vi "niFpgaFFTSimModelStreamingCoreWrapper.vi"(0 "real data in":fxp<+/-,16,1>, 1 "reset":bool, 5 "imaginary data in":fxp<+/-,16,1>, 7 "input valid":bool=TRUE, 12 "ready for output":bool=TRUE) -> (3 "data index":u16, 4 "real data out":fxp<+/-,32,16> format="%.21g", 6 "imaginary data out":fxp<+/-,32,16> format="%.21g", 8 "output valid":bool, 14 "ready for input":bool)   [LabVIEW 2017]
uses:
  <vilib>/rvi/Analysis/measure/FFT/simModelSupport/niFPGA FFT Streaming Sim Properties.ctl
  <vilib>/rvi/Analysis/measure/FFT/simModelSupport/niFPGA FFT Sim Stream Group Properties.ctl
  <vilib>/rvi/Analysis/measure/FFT/simModelSupport/niFPGA FFT Sim Types.ctl
  <vilib>/rvi/Analysis/measure/FFT/simModelSupport/niFpgaFFTSimArithmeticProperties.ctl
  <vilib>/rvi/Analysis/measure/FFT/simModelSupport/niFpgaFFTSimDfxp.ctl
  <vilib>/fxp/LVFixedPointQuantizationPolicyTypeDef.ctl
  <vilib>/rvi/Analysis/measure/FFT/XNode/niFpgaFFTButterflyDelays.ctl
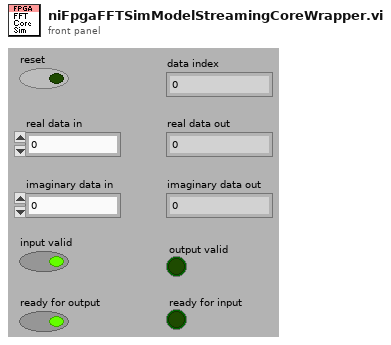
[diagram p1: front panel]
types:
  T1 = typedef "niFPGA FFT Streaming Sim Properties.ctl" = cluster{"scale factor":i32, "Group Settings":T2, "execution constants":cluster{"bitmask":u16, "K-16":i8}, "initial state":cluster{"iteration count":u16, "lty_count":u16, "idxv":bool, "os":bool}}
  T2 = typedef "niFPGA FFT Sim Stream Group Properties.ctl" = cluster{"Forward?":bool, "twiddle over 16?":bool, "number of stages":u8, "use pipeline registers":bool, "FFT fxp types":T3, "butterfly delays":T7}
  T3 = typedef "niFPGA FFT Sim Types.ctl" = cluster{"mult output type":T4, "internal type":T4, "twid type":T4, "sub output type":T4}
  T4 = typedef "niFpgaFFTSimArithmeticProperties.ctl" = cluster{"Output Type":T5, "Adapt To Source?":bool, "Rounding Mode":T6}
  T5 = typedef "niFpgaFFTSimDfxp.ctl" = cluster{"U64 Rep":u64, "Signed?":bool, "Word Length":i32, "Integer Word Length":i32}
  T6 = typedef "LVFixedPointQuantizationPolicyTypeDef.ctl" = enum32{"Truncate", "Round-Half-Up (Asymmetric)", "Round-Half-Even"}
  T7 = typedef "niFpgaFFTButterflyDelays.ctl" = cluster{"pre-scaling delay":u16, "post-scaling delay":u16, "boolean delay":u16}
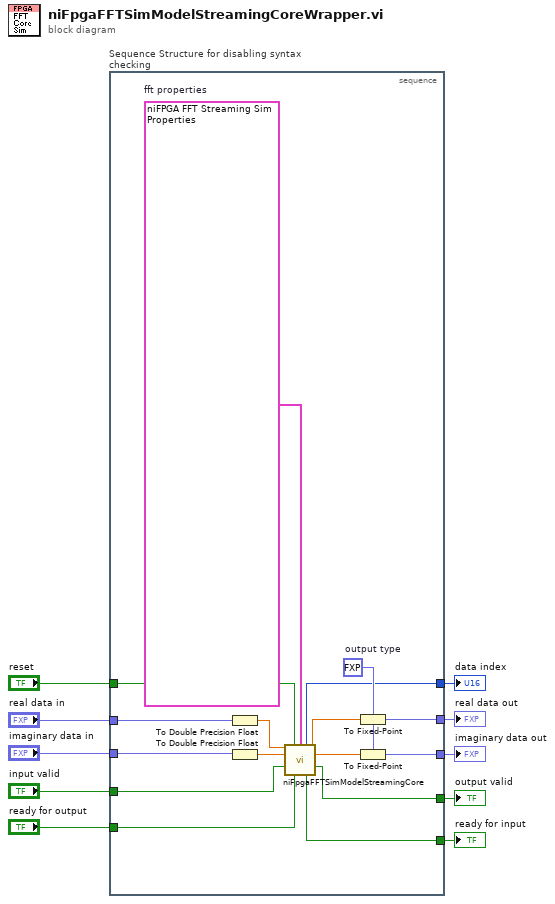
[diagram p0: block diagram]
diagram:
  n1 = stacked-sequence "Sequence Structure for disabling syntax checking" {
    tunnel: [w20] -> w10
    tunnel: [w19] -> w9
    tunnel: [w18] -> w8
    tunnel: [w17] -> w7
    tunnel: [w16] -> w6
    tunnel: "reset" -> [w15]
    tunnel: "real data in" -> [w14]
    tunnel: "imaginary data in" -> [w13]
    tunnel: "input valid" -> [w12]
    tunnel: "ready for output" -> [w11]
    frame #0 {
      w26 = T1 {"scale factor"=9, "Group Settings"={"Forward?"=FALSE, "twiddle over 16?"=FALSE, "number of stages"=0, "use pipeline registers"=FALSE, "FFT fxp types"={"mult output type"={"Output Type"={"U64 Rep"=0, "Signed?"=FALSE, "Word Length"=0, "Integer Word Length"=0}, "Adapt To Source?"=FALSE, "Rounding Mode"=enum."Truncate"}, "internal type"={"Output Type"={"U64 Rep"=0, "Signed?"=FALSE, "Word Length"=0, "Integer Word Length"=0}, "Adapt To Source?"=FALSE, "Rounding Mode"=enum."Truncate"}, "twid type"={"Output Type"={"U64 Rep"=0, "Signed?"=FALSE, "Word Length"=0, "Integer Word Length"=0}, "Adapt To Source?"=FALSE, "Rounding Mode"=enum."Truncate"}, "sub output type"={"Output Type"={"U64 Rep"=0, "Signed?"=FALSE, "Word Length"=0, "Integer Word Length"=0}, "Adapt To Source?"=FALSE, "Rounding Mode"=enum."Truncate"}}, "butterfly delays"={"pre-scaling delay"=0, "post-scaling delay"=0, "boolean delay"=0}}, "execution constants"={"bitmask"=255, "K-16"=-8}, "initial state"={"iteration count"=128, "lty_count"=412, "idxv"=FALSE, "os"=FALSE}}  # fft properties
      w25 = fxp<+/-,32,16> 0.0  # output type
      n2 = To Double Precision Float(number=w14) -> (double precision float=w22:dbl)
      n3 = To Double Precision Float(number=w13) -> (double precision float=w21:dbl)
      n4 = call <vilib>:"niFpgaFFTSimModelStreamingCore.vi"("real data in"=w22, "reset"=w15, "streaming settings"=w26, "imaginary data in"=w21, "input valid"=w12, "ready for output"=w11) -> ("data index"=w20:u16, "real data out"=w23:dbl, "imaginary data out"=w24:dbl, "output valid"=w17:bool, "ready for input"=w16:bool)  [unwired: 5 out]
      n5 = To Fixed-Point(fixed-point type=w25, number=w23) -> (fixed-point=w19:fxp<+/-,32,16>)
      n6 = To Fixed-Point(fixed-point type=w25, number=w24) -> (fixed-point=w18:fxp<+/-,32,16>)
    }
  }
  "ready for input" <- w6
  "output valid" <- w7
  "real data out" <- w9
  "imaginary data out" <- w8
  "data index" <- w10
